vi "Continuity_SMUResistanceTest.vi"(7 "Published Data Id":T2, 9 "DCPower_Parameters":T1={"Output"=enum."DC Voltage", "Current_range"=0.0, "Current"=0.0, "Voltage_range"=0.0, "Voltage"=0.0, "Aperture_time"=0.0, "Source Delay"=0.0, "Sense"=1008} {"Source Delay" format="%.6p"; "Sense" items=["Local"=1008, "Remote"=1009]; "Aperture_time" format="%.6p"; "Current_range" format="%.6p"; "Current" format="%.6p"; "Voltage_range" format="%.6p"; "Voltage" format="%.6p"}, 10 "Pins":T3[](array[typedef]), 11 "Semiconductor Module Context":T4) -> (0 "error out":errorcluster)   [LabVIEW 2023, in "Continuity.lvlib"]
doc: "Measures the resistance using an SMU channel in order to perform simple Continuity Test"
uses:
  Continuity.lvlib
  <vilib>/NI_TestStand_SemiconductorModule/NI_TestStand_Semiconductor_Module.lvlibp/PinMap/General/SemiconductorModuleContext.ctl
  <vilib>/NI_TestStand_SemiconductorModule/NI_TestStand_Semiconductor_Module.lvlibp/PinMap/TagProvider/TSM_Pin.ctl
  <vilib>/NI_TestStand_SemiconductorModule/NI_TestStand_Semiconductor_Module.lvlibp/PinMap/TagProvider/TSM_PublishedDataId.ctl
  ResourceHandling/TypeDefs/RH_DCPower_Parameters.ctl
  <vilib>/NI_TestStand_SemiconductorModule/NI_TestStand_Semiconductor_Module.lvlibp/PinMap/DC Power/PinsToNIDCPowerSessions.vi
  <vilib>/NI_TestStand_SemiconductorModule/NI_TestStand_Semiconductor_Module.lvlibp/PinMap/General/Publish/PublishDataPerSiteDoubleScalar.vi
  ResourceHandling/ResourceHandling.lvlib
  <vilib>/NI_TestStand_SemiconductorModule/NI_TestStand_Semiconductor_Module.lvlibp
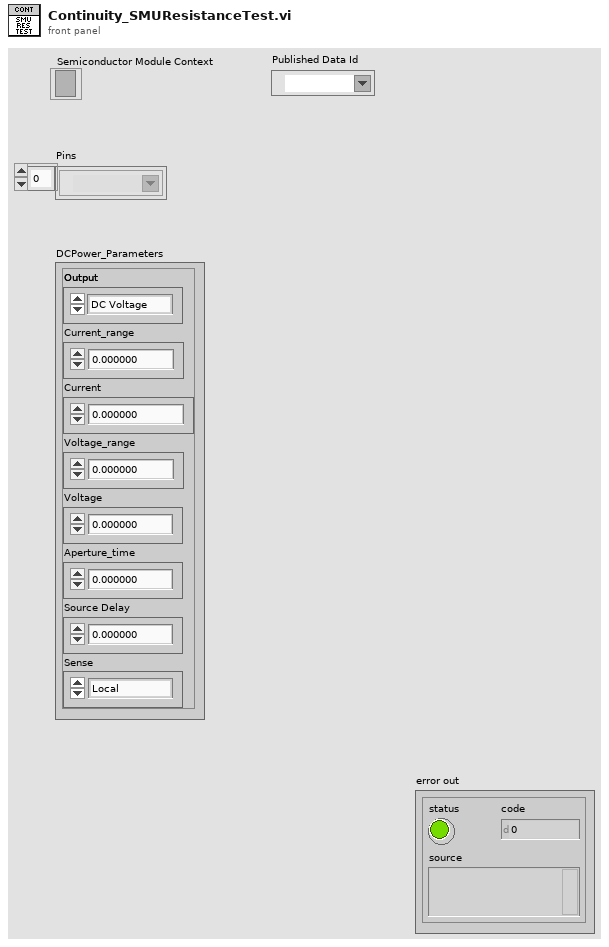
[diagram p1: front panel]
types:
  T1 = typedef "ResourceHandling.lvlib/RH_DCPower_Parameters.ctl" = cluster{"Output":enum16{"DC Voltage", "DC Current"}, "Current_range":dbl, "Current":dbl, "Voltage_range":dbl, "Voltage":dbl, "Aperture_time":dbl, "Source Delay":dbl, "Sense":i32}
  T2 = typedef "NI_TestStand_Semiconductor_Module.lvlibp/TSM_PublishedDataId.ctl" = tag
  T3 = typedef "NI_TestStand_Semiconductor_Module.lvlibp/TSM_Pin.ctl" = tag
  T4 = typedef "NI_TestStand_Semiconductor_Module.lvlibp/SemiconductorModuleContext.ctl" = refnum<k7>
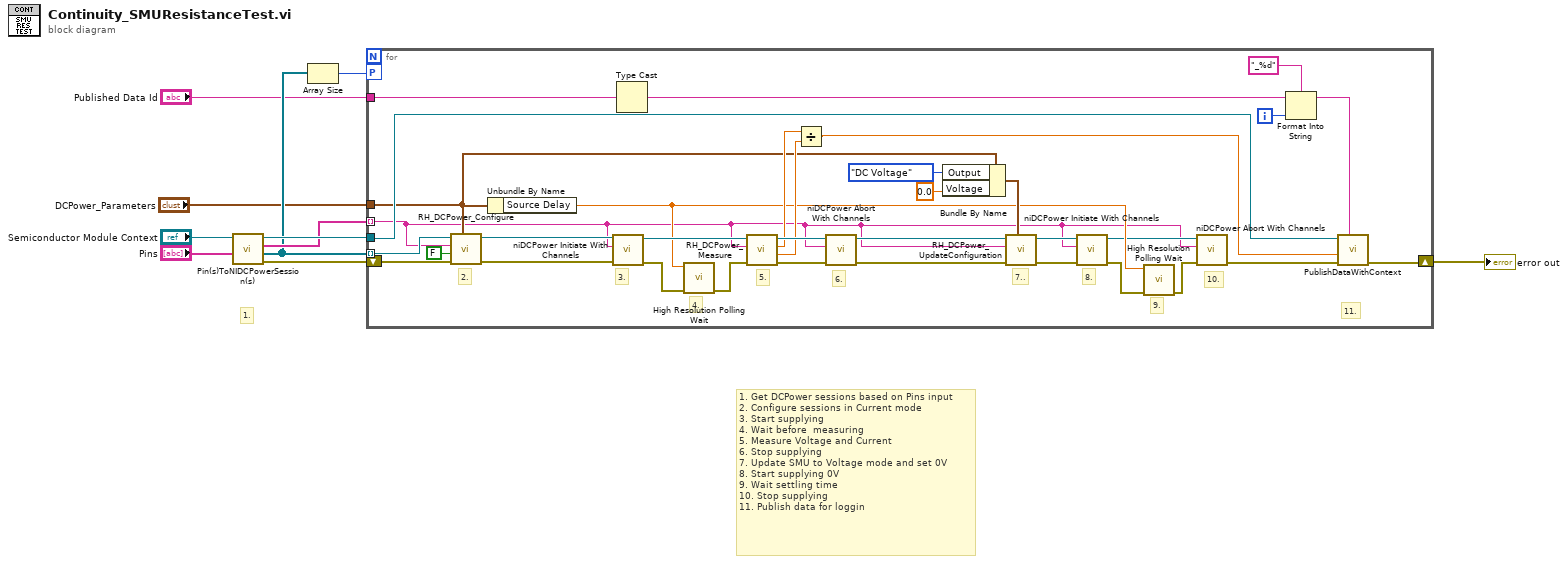
[diagram p0: block diagram]
diagram:
  # "1. Get DCPower sessions based on Pins input\n2. Configure sessions in Current mode\n3. Start supplying\n4. Wait before  measuring\n5. Measure Voltage and Current\n6. Stop supplying\n7. Update SMU to Voltage mode and set 0V\n8. Start supplying 0V\n9. Wait settling time\n10. Stop supplying\n11. Publish data for loggin"
  # "1."
  n1 = call-poly <vilib>:"Pin(s)ToNIDCPowerSession(s).vi"("Pins"="Pins", "Semiconductor Module Context"="Semiconductor Module Context") -> ("error out"=w7:errorcluster, "Instrument Sessions"=w4:refnum<k15>[], "Channel Strings"=w6:string[], "Semiconductor Module Context Out"=w8:T4)  [unwired: 5 in, 1 out]
  n2 = Array Size(array=w4) -> (size(s)=w5:i32)
  n3 = for {
    tunnel: w8 -> [w36]
    shift-right: [w29] -> w3
    shift-left: w7 -> [w44]
    tunnel: w6 -> [w15] mode=indexing
    tunnel: w4 -> [w43] mode=indexing
    workers-P: w5 -> [_]
    tunnel: "DCPower_Parameters" -> [w26]
    tunnel: "Published Data Id" -> [w30]
    i -> [w12]
    # "11."
    # "10."
    # "9."
    # "8."
    # "7.."
    # "6."
    # "5."
    # "4."
    # "3."
    # "2."
    n4 = call "RH_DCPower_Configure.vi"("DCPower_Parameters"=w26, "error in (no error)"=w44, "trigger out?"=FALSE, "channel name"=w15, "DCPower Session In"=w43) -> ("error out"=w40:errorcluster, "DCPower Session Out"=w41:refnum<k15>)  [unwired: 5 in]
    n5 = Unbundle By Name(w26) -> ("Source Delay"=w19:dbl)
    n6 = call <instrlib>:"niDCPower Initiate With Channels.vi"("error in (no error)"=w40, "channel name"=w15, "instrument handle"=w41) -> ("error out"=w39:errorcluster, "instrument handle out"=w38:refnum<k15>)  [unwired: 7 in]
    n7 = Type Cast(x=w30) -> (*(type *) &x=w14:string)  [unwired: 1 in]
    n8 = call <vilib>:"High Resolution Polling Wait.vi"("error in (no error)"=w39, "seconds to wait"=w19) -> ("error out"=w37:errorcluster)  [unwired: 9 in]
    n9 = call "RH_DCPower_Measure.vi"("error in (no error)"=w37, "channel name"=w15, "DCPower Session In"=w38) -> ("error out"=w35:errorcluster, "Current"=w32:dbl, "Voltage"=w33:dbl, "DCPower Session Out"=w34:refnum<k15>)  [unwired: 5 in]
    n10 = Divide(x=w33, y=w32) -> (x/y=w31:dbl)
    n11 = call <instrlib>:"niDCPower Abort With Channels.vi"("error in (no error)"=w35, "channel name"=w15, "instrument handle"=w34) -> ("error out"=w28:errorcluster, "instrument handle out"=w27:refnum<k15>)  [unwired: 7 in]
    n12 = Bundle By Name(cluster=w26, "Output"=enum16{"DC Voltage", "DC Current"}."DC Voltage", "Voltage"=0.0) -> (w25:T1)
    n13 = call "RH_DCPower_UpdateConfiguration.vi"("DCPower_Parameters"=w25, "error in (no error)"=w28, "channel name"=w15, "DCPower Session In"=w27) -> ("error out"=w22:errorcluster, "DCPower Session Out"=w21:refnum<k15>)  [unwired: 6 in]
    n14 = call <instrlib>:"niDCPower Initiate With Channels.vi"("error in (no error)"=w22, "channel name"=w15, "instrument handle"=w21) -> ("error out"=w20:errorcluster, "instrument handle out"=w16:refnum<k15>)  [unwired: 7 in]
    n15 = call <vilib>:"High Resolution Polling Wait.vi"("error in (no error)"=w20, "seconds to wait"=w19) -> ("error out"=w18:errorcluster)  [unwired: 9 in]
    n16 = call <instrlib>:"niDCPower Abort With Channels.vi"("error in (no error)"=w18, "channel name"=w15, "instrument handle"=w16) -> ("error out"=w17:errorcluster)  [unwired: 7 in, 1 out]
    n17 = Format Into String(format string="_%d", initial string=w14, w12) -> (resulting string=w11:string)  [unwired: 1 in, 1 out]
    n18 = call-poly <vilib>:"PublishDataWithContext.vi"("Published Data Id"=w11, "error in (no error)"=w17, "Data In"=w31, "Semiconductor Module Context"=w36) -> ("error out"=w29:errorcluster)  [unwired: 6 in, 1 out]
  }
  "error out" <- w3
